vi "use_num_add.vi"() -> ()   [LabVIEW 2018]
uses:
  float_add.vi
  posit.lvlib
panel:
  out "y":sgl
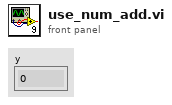
[diagram p1: front panel]
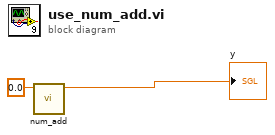
[diagram p0: block diagram]
diagram:
  n1 = call-poly "num_add.vi"("x"=sgl 0.0) -> ("y"=→"y":sgl)  [unwired: 10 in]
